vi "CoMP-S Rotation calculate.vi"(9 "New Value":dbl, 10 "Old Value":dbl) -> (2 "Direction":bool=TRUE, 3 "steps":i32, 4 "Degrees":i32, 5 "rotate direction":string)   [LabVIEW 2014]
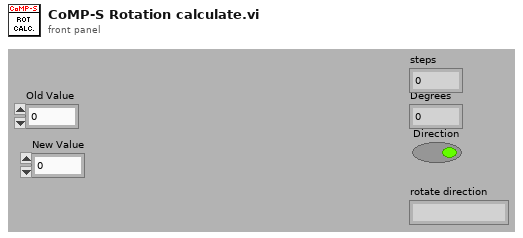
[diagram p1: front panel]
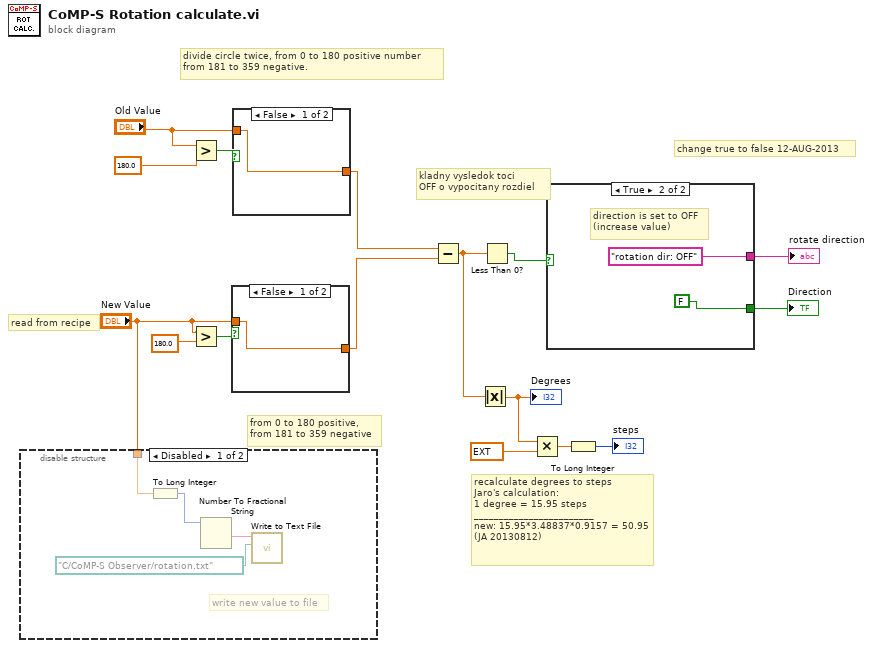
[diagram p0: block diagram]
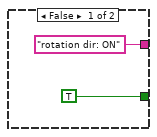
[diagram p3: hidden frame]
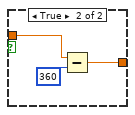
[diagram p4: hidden frame]
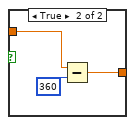
[diagram p5: hidden frame]
diagram:
  # "change true to false 12-AUG-2013"
  # "recalculate degrees to steps\nJaro's calculation:\n1 degree = 15.95 steps\n________________________\nnew: 15.95*3.48837*0.9157 = 50.95\n(JA 20130812)"
  # "from 0 to 180 positive, \nfrom 181 to 359 negative"
  # "divide circle twice, from 0 to 180 positive number\nfrom 181 to 359 negative."
  # "kladny vysledok toci\nOFF o vypocitany rozdiel"
  # "read from recipe"
  n1 = disable-structure shown="Disabled" {
    disable-tunnel: "New Value" -> [w20 _]
    frame Disabled {
      # "write new value to file"
      n2 = To Long Integer(number=w20) -> (32bit integer=w18:i32)
      n3 = Number To Fractional String(number=w18) -> (F-format string=w19:string)  [unwired: 3 in]
      n4 = call "Write to Text File.vi"("file path (use dialog)"=path "C:/CoMP-S Observer/rotation.txt", "text"=w19) -> ()  [unwired: 9 in, 1 out]
    }
    frame Enabled {
    }
  }
  n5 = Greater?(x="Old Value", y=180.0) -> (0:w13:bool)
  n6 = Greater?(x="New Value", y=180.0) -> (0:w12:bool)
  n7 = case shown="False" w12 {
    tunnel: "New Value" -> [w21 w23]
    tunnel: [w21 w22] -> w1
    frame False {
    }
    frame True {
      n8 = Subtract(x=w23, y=360) -> (x-y=w22:dbl)
    }
  }
  n9 = case shown="False" w13 {
    tunnel: [w25 w27] -> w11
    tunnel: "Old Value" -> [w25 w26]
    frame False {
    }
    frame True {
      n10 = Subtract(x=w26, y=360) -> (x-y=w27:dbl)
    }
  }
  n11 = Subtract(x=w11, y=w1) -> (x-y=w7:dbl)
  n12 = Absolute Value(x=w7) -> (abs(x)=w6:dbl)
  "Degrees" <- w6
  n13 = Less Than 0?(x=w7) -> (x < 0?=w10:bool)
  n14 = Multiply(x=w6, y=ext 50.95) -> (x*y=w4:ext)
  n15 = case shown="True" w10 {
    tunnel: ["rotation dir: ON" "rotation dir: OFF"] -> w9
    tunnel: [TRUE FALSE] -> w8
    frame False {
    }
    frame True {
      # "direction is set to OFF\n(increase value)"
    }
  }
  "rotate direction" <- w9
  "Direction" <- w8
  n16 = To Long Integer(number=w4) -> (32bit integer=→"steps":i32)
